vi "Test App Error Handler is Configured as App Process Error Handler for Process Added after Setting Error Handler.vi"(8 "error in (no error)":errorcluster, 11 "Rig Test In":refnum<class "Application Test.lvclass">) -> (0 "error out":errorcluster, 3 "Rig Test Out":refnum<class "Application Test.lvclass">)   [LabVIEW 2020, in "Application Test.lvclass"]
uses:
  Application Test.lvclass
  C:/Program Files (x86)/National Instruments/LabVIEW 2020/vi.lib/Asteme/LUnit/Test Case.lvclass
  Mock Error Handler/Mock Error Handler.lvclass
  C:/Users/anton/Documents/GitHub/Triarc-Framework/source/Framework/Error Handler Interface/Error Handler Interface.lvclass
  Mock Process/Mock Process.lvclass
  C:/Users/anton/Documents/GitHub/Triarc-Framework/source/Framework/Process/Process.lvclass
  Framework/Error Handler Interface/Error Handler Interface.lvclass
  Framework/Process/Process.lvclass/Process.ctl
  Framework/Application/Application.lvclass/Application.ctl
  <vilib>/Asteme/LUnit/Test Case.lvclass/Test Case.ctl
  <vilib>/Asteme/LUnit/LUnit Assertion Result.lvclass/LUnit Assertion Result.ctl
  Framework/Process/Public/Lifecycle/Get Lifecycle State.vi
  Framework/Process/Protected/Messaging/Enqueue Message.vi
  <vilib>/Utility/error.llb/Clear Errors.vi
  Framework/Process/Protected/SubVIs/Set Context.vi
  Framework/Application/Private/Add Process to Map.vi
  Framework/Process/Private/SubVIs/Wait for finish.vi
  Framework/Process/Private/SubVIs/Set Lifecycle State.vi
  <vilib>/Asteme/LUnit/Palette/Pass.vi
  <vilib>/Asteme/LUnit/Palette/Fail.vi
  <vilib>/Asteme/LUnit/Variant to string.vi
  <vilib>/Asteme/LUnit/Set Assertion Type.vi
  <vilib>/AdvancedString/1D String Array to Delimited String.vi
  <vilib>/Asteme/LUnit/Add test result.vi
  <vilib>/Asteme/LUnit/LUnit Write Passed.vi
  <vilib>/Asteme/LUnit/LUnit Get Test Case.vi
  <vilib>/Asteme/LUnit/LUnit Write Message.vi
  <vilib>/Asteme/LUnit/LUnit Write Description.vi
  <vilib>/Asteme/LUnit/LUnit Write Assertion Type.vi
  <vilib>/Asteme/LUnit/Read Test Case Name.vi
  Framework/Application/Application.lvclass
  <vilib>/Utility/error.llb/Error Cluster From Error Code.vi
  <vilib>/Asteme/LUnit/Assertion Result/LUnit Get Test Name.vi
  <vilib>/Utility/Data Type/Get Type Information.vi
  <vilib>/Utility/LVClass/Get LV Class Name.vi
  Framework/Process/Process.lvclass
  <vilib>/Asteme/LUnit/LUnit Assertion Result.lvclass
  C:/Users/anton/Documents/GitHub/Triarc-Framework/source/Framework/Base/Base.lvclass
  C:/Users/anton/Documents/GitHub/Triarc-Framework/source/Framework/Application/Application.lvclass
  <vilib>/Asteme/LUnit/Test Case.lvclass
  C:/Users/anton/Documents/GitHub/Triarc-Framework/source/Framework Test/Mock Error Handler/Mock Error Handler.lvclass
  C:/Users/anton/Documents/GitHub/Triarc-Framework/source/Framework Test/Mock Process/Mock Process.lvclass
  C:/Users/anton/Documents/GitHub/Triarc-Framework/source/Framework/Helper Loop/Helper Loop.lvclass
  C:/Users/anton/Documents/GitHub/Triarc-Framework/source/Framework Test/Process Test/Process Test.lvclass
  C:/Users/anton/Documents/GitHub/Triarc-Framework/source/Framework Test/Base Class Test/Base Test.lvclass
  C:/Users/anton/Documents/GitHub/Triarc-Framework/source/Framework Test/Application Test/Application Test.lvclass
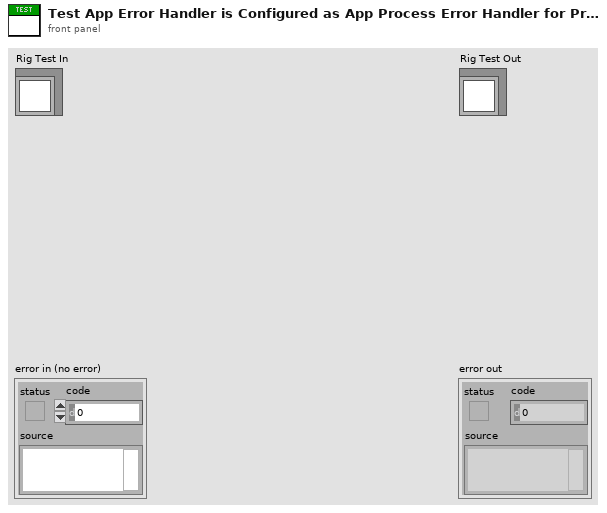
[diagram p1: front panel]
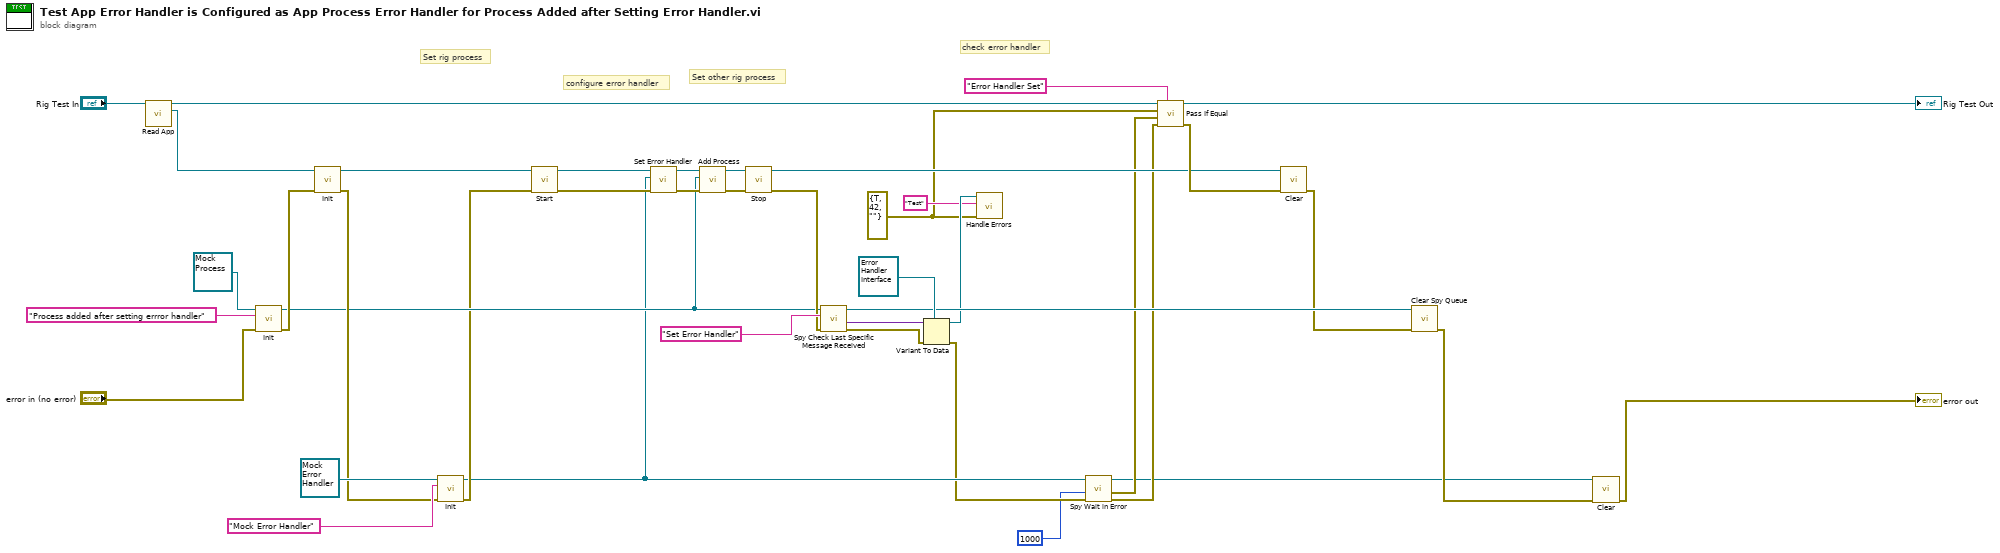
[diagram p0: block diagram]
diagram:
  w7 = errorcluster {"status"=TRUE, "code"=42, "source"=""} ("error in (no error)")
  # "check error handler"
  # "Set other rig process"
  # "configure error handler"
  # "Set rig process"
  n1 = call "Read App.vi"("Application Test In"="Rig Test In") -> ("App out"=w40:refnum<class "Application.lvclass">, "Application Test Out"=w36:refnum<class "Application Test.lvclass">)  [unwired: 8 in, 1 out]
  n2 = call-dynamic "Init.vi"("error in (no error)"="error in (no error)", "Name"="Process added after setting errror handler", "Mock Process In"=refnum<class "Mock Process.lvclass"> refnum ("Mock Process.lvclass")) -> ("error out"=w30:errorcluster, "Mock Process Out"=w10:refnum<class "Mock Process.lvclass">)  [unwired: 7 in]
  n3 = call-dynamic "Init.vi"("error in (no error)"=w30, "Process In"=w40) -> ("error out"=w29:errorcluster, "Process Out"=w39:refnum<class "Application.lvclass">)  [unwired: 8 in]
  n4 = call-dynamic "Init.vi"("error in (no error)"=w29, "Name"="Mock Error Handler", "Mock Error Handler In"=refnum<class "Mock Error Handler.lvclass"> refnum ("Mock Error Handler.lvclass")) -> ("error out"=w5:errorcluster, "Mock Error Handler Out"=w4:refnum<class "Mock Error Handler.lvclass">)  [unwired: 7 in]
  n5 = call "Start.vi"("error in (no error)"=w5, "Process In"=w39) -> ("error out"=w17:errorcluster, "Process Out"=w18:refnum<class "Application.lvclass">)  [unwired: 8 in]
  n6 = call "Set Error Handler.vi"("error in (no error)"=w17, "Error Handler"=w4, "Process In"=w18) -> ("error out"=w13:errorcluster, "Process Out"=w14:refnum<class "Application.lvclass">)  [unwired: 7 in]
  n7 = call "Add Process.vi"("error in (no error)"=w13, "Process"=w10, "Rig In"=w14) -> ("error out"=w11:errorcluster, "Rig Out"=w12:refnum<class "Application.lvclass">)  [unwired: 7 in]
  n8 = call "Stop.vi"("error in (no error)"=w11, "Process In"=w12) -> ("error out"=w24:errorcluster, "Process Out"=w26:refnum<class "Application.lvclass">)  [unwired: 7 in, 1 out]
  n9 = call "Spy Check Last Specific Message Received.vi"("error in (no error)"=w24, "Specific Call"="Set Error Handler", "Mock Rig Process In"=w10) -> ("error out"=w19:errorcluster, "Message Data"=w23:variant, "Mock Rig Process Out"=w21:refnum<class "Mock Process.lvclass">)  [unwired: 5 in, 1 out]
  n10 = Variant To Data(error in=w19, type=refnum<class "Error Handler Interface.lvclass"> refnum ("Process In"), Variant=w23) -> (data=w20:refnum<class "Error Handler Interface.lvclass">, error out=w2:errorcluster)
  n11 = call-dynamic "Handle Errors.vi"("error in (no error)"=w7, "Location"="Test", "Error Handler Interface In"=w20) -> ()  [unwired: 7 in, 2 out]
  n12 = call "Spy Wait in Error.vi"("error in (no error)"=w2, "timeout in ms (-1)"=1000, "Mock Error Handler In"=w4) -> ("error out"=w8:errorcluster, "Errors"=w6:errorcluster, "Mock Error Handler Out"=w3:refnum<class "Mock Error Handler.lvclass">)  [unwired: 4 in, 2 out]
  n13 = call <vilib>:"Pass If Equal.vi"("Description"="Error Handler Set", "error in (no error)"=w8, "Actual"=w6, "Expected"=w7, "Test Case In"=w36) -> ("error out"=w28:errorcluster, "Test Case Out"=→"Rig Test Out":refnum<class "Application Test.lvclass">)  [unwired: 5 in]
  n14 = call-dynamic "Clear.vi"("error in (no error)"=w28, "Application In"=w26) -> ("error out"=w16:errorcluster)  [unwired: 8 in, 1 out]
  n15 = call-dynamic "Clear Spy Queue.vi"("error in (no error)"=w16, "Mock Process In"=w21) -> ("error out"=w15:errorcluster)  [unwired: 8 in, 1 out]
  n16 = call-dynamic "Clear.vi"("error in (no error)"=w15, "Mock Process In"=w3) -> ("error out"=→"error out":errorcluster)  [unwired: 8 in, 1 out]
